vi "m100RecipeToExcelNew.vi"() -> ()   [LabVIEW 2012]
uses:
  <vilib>/addons/database/Auxilliary.llb/DB Tools Cursor Type.ctl
  <vilib>/Utility/NIReport.llb/NI_report.lvclass
  <vilib>/addons/database/Connection.llb/DB Tools Open Connec (Path).vi
  <vilib>/addons/database/Connection.llb/Conn Execute.vi
  <vilib>/addons/database/Recordset.llb/Rec Fetch Recordset Data (R).vi
  <vilib>/addons/database/Recordset.llb/Rec Destroy - Connection.vi
  <vilib>/Utility/NIReport.llb/Append Text Table to Report (wrap).vi
  <vilib>/addons/database/_DB Variant To Data/Database Variant To Data.xnode
  <vilib>/Utility/NIReport.llb/Excel/NI_Excel.lvclass
  <vilib>/addons/database/NI_Database_API.lvlib
panel:
  in  "template (empty)":path=path "O:/Monitor/Recipe/PTSE/Module_Recipe Mapping Table.xls"
  out "appended path":path
  out "error out 4":errorcluster
  out "recordset data":variant[][](array[variant])
  out "error out":errorcluster
  in  "Report Template":path=path "O:/Monitor/Report/Module_Recipe Mapping Table.xls"
  in  "Table Control":string[][](table)
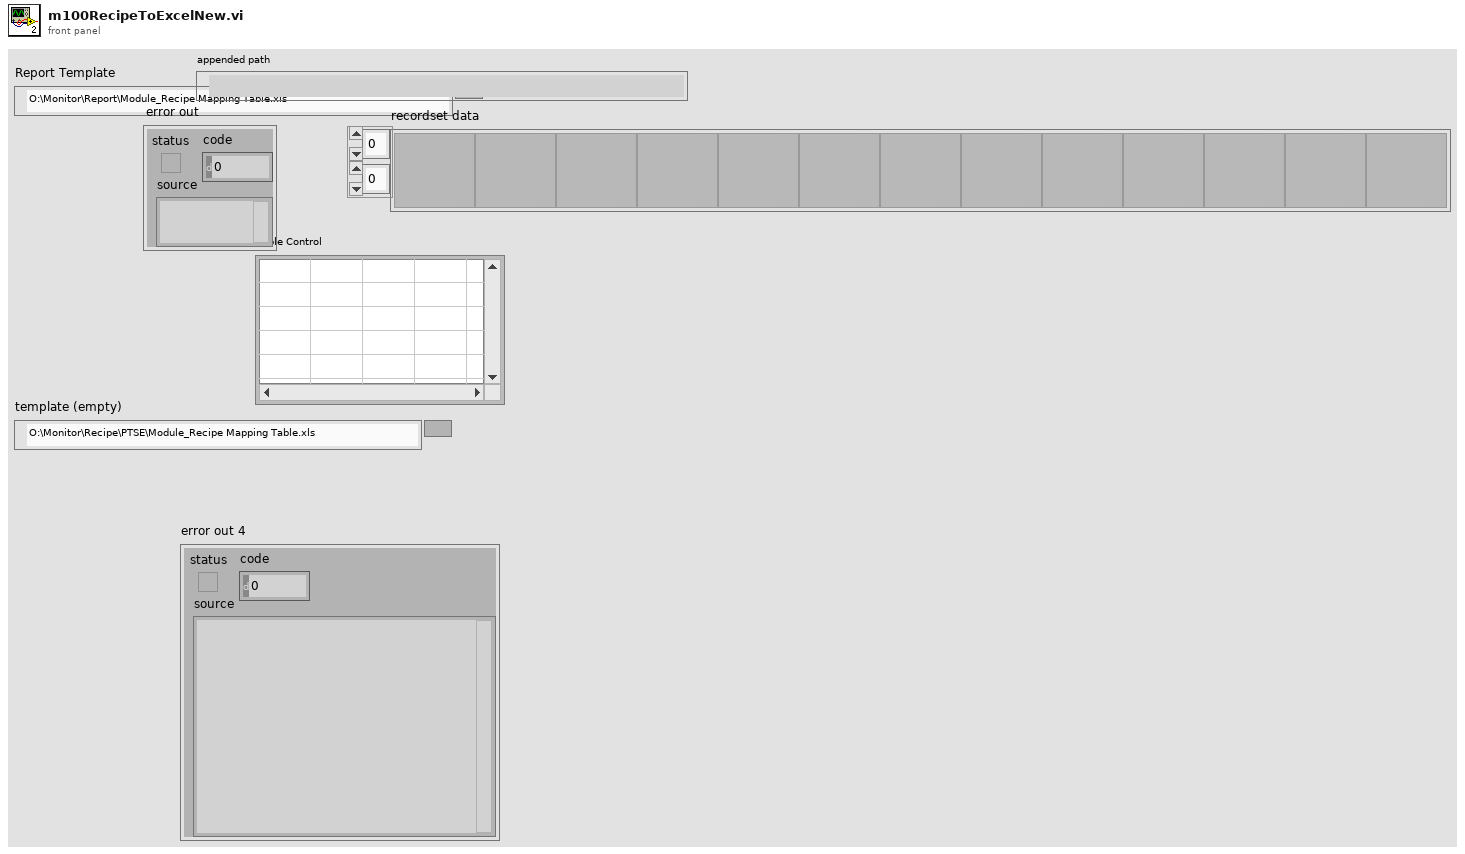
[diagram p1: front panel]
types:
  T1 = typedef "NI_Database_API.lvlib/DB Tools Cursor Type.ctl" = enum16{"forward-only", "keyset", "dynamic", "static"}
  T2 = typedef "NI_Database_API.lvlib/Conn ObjectReference.ctl" = refnum<k1>
  T3 = typedef "NI_Database_API.lvlib/Rec ObjectReference.ctl" = refnum<k1>
  T4 = enum16{"Standard Report", "HTML", "Word", "Excel"}
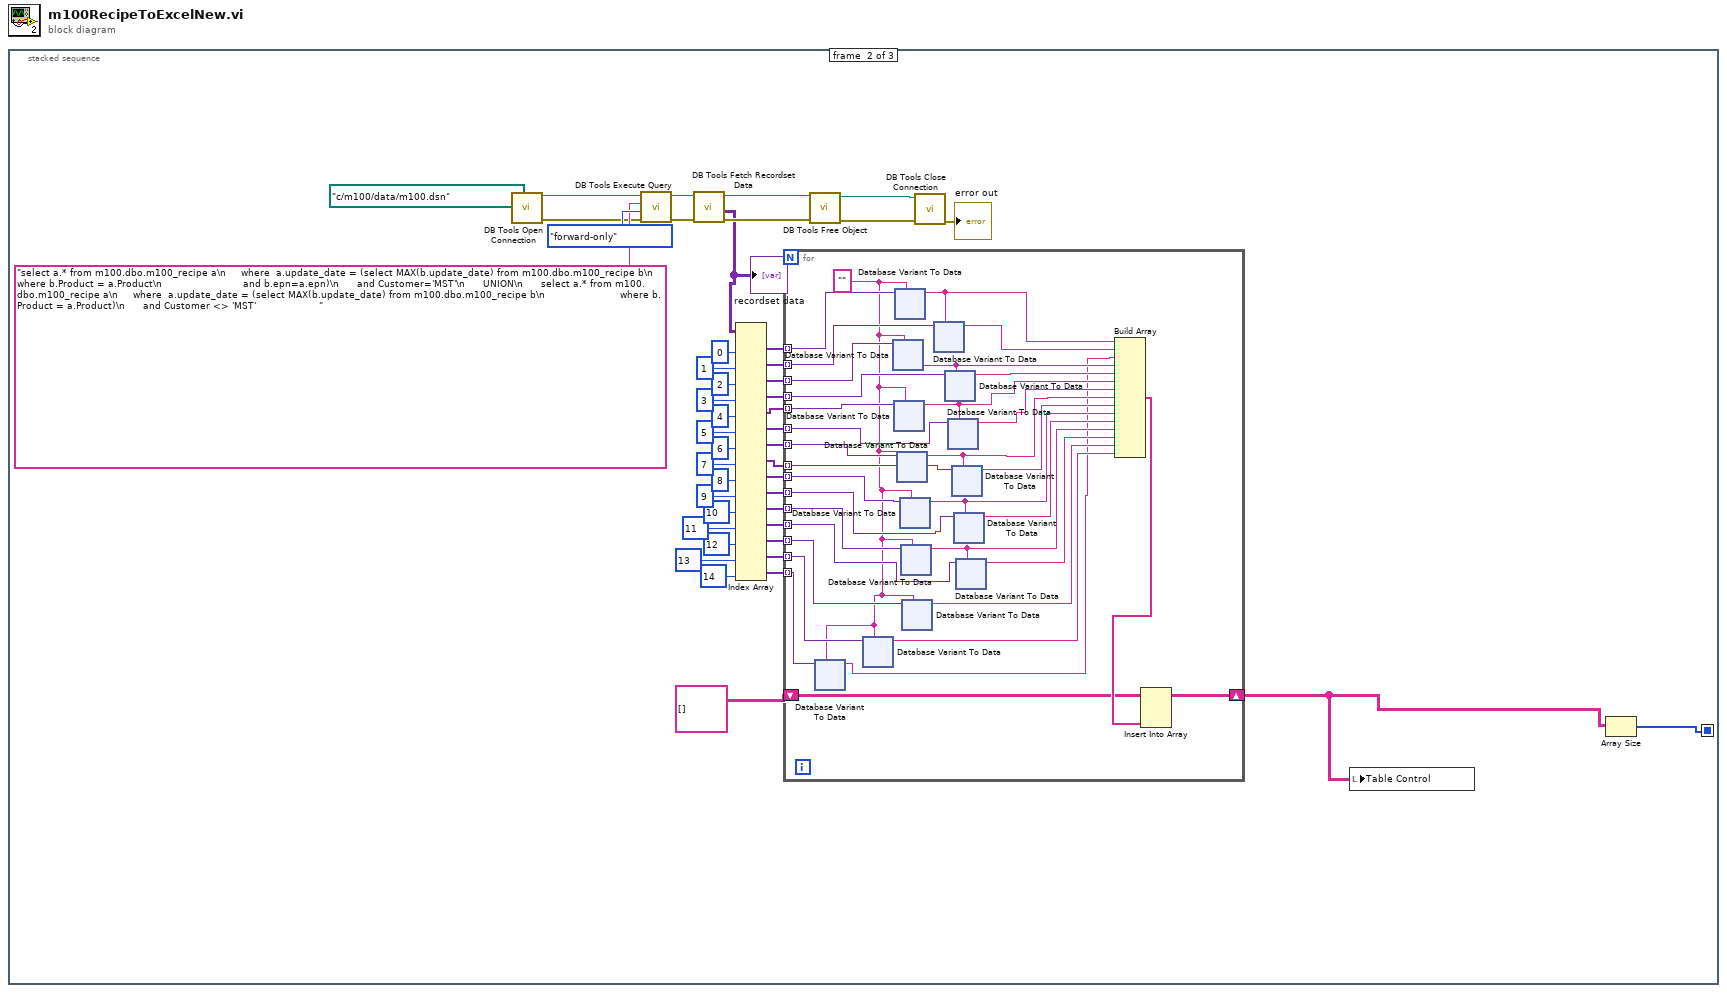
[diagram p0: block diagram]
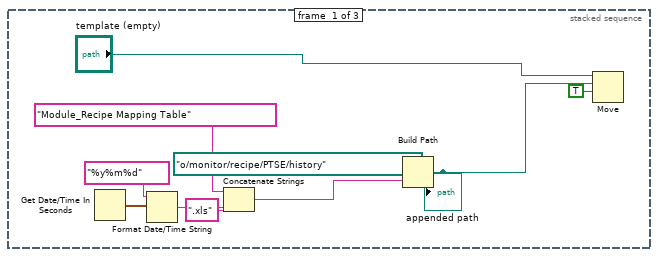
[diagram p2: hidden frame]
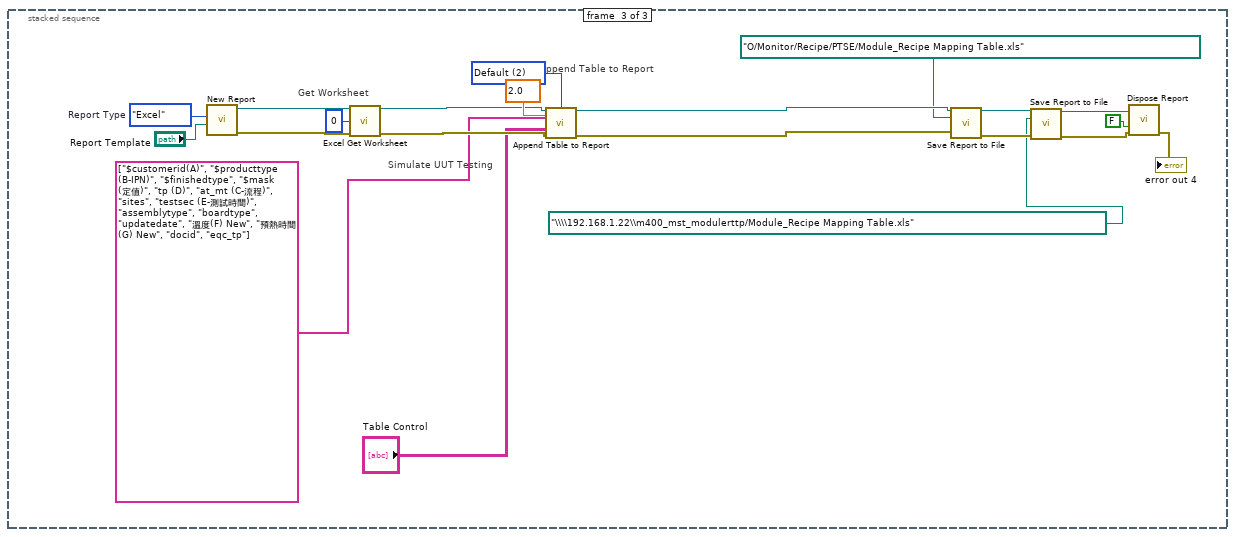
[diagram p3: hidden frame]
diagram:
  n1 = stacked-sequence {
    seq-local: [_ w56 _] -> [_ _ _]
    frame #0 {
      n2 = Get Date/Time In Seconds() -> (seconds since 1Jan1904=w8:timestamp)
      n3 = Format Date/Time String(time format string (%c)="%y%m%d", seconds (now)=w8) -> (date/time string=w6:string)  [unwired: 1 in]
      n4 = Concatenate Strings("Module_Recipe Mapping Table" ("string"), w6, ".xls" ("string")) -> (w9:string)
      n5 = Build Path(base path=path "o:/monitor/recipe/PTSE/history", name or relative path=w9) -> (appended path=w3:path)
      "appended path" <- w3
      n6 = Move(source path="template (empty)", 9:TRUE ("overwrite (F)"), 10:w3) -> ()  [unwired: 2 in, 3 out]
    }
    frame #1 {
      n7 = call-poly <vilib>:"DB Tools Open Connection.vi"("connection information"=path "c:/m100/data/m100.dsn") -> ("error out"=w23:errorcluster, "connection reference"=w24:T2)  [unwired: 7 in]
      n8 = call-poly <vilib>:"DB Tools Execute Query.vi"("error in (no error)"=w23, "cursor type"=DB_Tools_Cursor_Type."forward-only", "SQL query"="select a.* from m100.dbo.m100_recipe a\n     where  a.update_date = (select MAX(b.update_date) from m100.dbo.m100_recipe b\n                         where b.Product = a.Product\n                           and b.epn=a.epn)\n      and Customer='MST'\n      UNION\n      select a.* from m100.dbo.m100_recipe a\n     where  a.update_date = (select MAX(b.update_date) from m100.dbo.m100_recipe b\n                         where b.Product = a.Product)\n      and Customer <> 'MST'                     ", "connection reference"=w24) -> ("error out"=w55:errorcluster, "recordset reference"=w54:T3)  [unwired: 4 in]
      n9 = call-poly <vilib>:"DB Tools Fetch Recordset Data.vi"("error in (no error)"=w55, "recordset reference"=w54) -> ("error out"=w52:errorcluster, "recordset data"=w50:variant[][], "recordset reference out"=w53:T3)  [unwired: 3 in]
      "recordset data" <- w50
      n10 = Index Array(array=w50, index (col) #1=0 ("disabled index (col)"), index (col) #2=1 ("index (col)"), index (col) #3=2 ("index (col)"), index (col) #4=3 ("index (col)"), index (col) #5=4 ("index (col)"), index (col) #6=5 ("index (col)"), index (col) #7=6 ("index (col)"), index (col) #8=7 ("index (col)"), index (col) #9=8 ("index (col)"), index (col) #10=9 ("index (col)"), index (col) #11=10 ("index (col)"), index (col) #12=11 ("index (col)"), index (col) #13=12 ("index (col)"), index (col) #14=13 ("index (col)"), index (col) #15=14 ("index (col)")) -> (element #1=w47:variant[], element #2=w46:variant[], element #3=w45:variant[], element #4=w34:variant[], element #5=w33:variant[], element #6=w32:variant[], element #7=w31:variant[], element #8=w30:variant[], element #9=w29:variant[], element #10=w28:variant[], element #11=w27:variant[], element #12=w26:variant[], element #13=w17:variant[], element #14=w13:variant[], element #15=w11:variant[])  [unwired: 15 in]
      n11 = for {
        tunnel: w47 -> [w90] mode=indexing
        tunnel: w46 -> [w89] mode=indexing
        tunnel: w45 -> [w88] mode=indexing
        tunnel: w34 -> [w87] mode=indexing
        tunnel: w33 -> [w84] mode=indexing
        tunnel: w32 -> [w82] mode=indexing
        tunnel: w31 -> [w80] mode=indexing
        tunnel: w30 -> [w77] mode=indexing
        tunnel: w29 -> [w76] mode=indexing
        tunnel: w28 -> [w75] mode=indexing
        tunnel: w27 -> [w72] mode=indexing
        tunnel: w26 -> [w71] mode=indexing
        tunnel: w17 -> [w68] mode=indexing
        shift-right: [w65] -> w15
        shift-left: string[][] [] ("array") -> [w64]
        tunnel: w13 -> [w63] mode=indexing
        tunnel: w11 -> [w61] mode=indexing
        w60 = ""
        n12 = xnode "Database Variant To Data"("database variant"=w61, "type"=w60) -> ("data"=w57:string)  [unwired: 1 in, 1 out]
        n13 = xnode "Database Variant To Data"("database variant"=w63, "type"=w60) -> ("data"=w62:string)  [unwired: 1 in, 1 out]
        n14 = xnode "Database Variant To Data"("database variant"=w88, "type"=w60) -> ("data"=w86:string)  [unwired: 1 in, 1 out]
        n15 = xnode "Database Variant To Data"("database variant"=w84, "type"=w60) -> ("data"=w83:string)  [unwired: 1 in, 1 out]
        n16 = xnode "Database Variant To Data"("database variant"=w90, "type"=w60) -> ("data"=w59:string)  [unwired: 1 in, 1 out]
        n17 = xnode "Database Variant To Data"("database variant"=w80, "type"=w60) -> ("data"=w79:string)  [unwired: 1 in, 1 out]
        n18 = xnode "Database Variant To Data"("database variant"=w76, "type"=w60) -> ("data"=w74:string)  [unwired: 1 in, 1 out]
        n19 = xnode "Database Variant To Data"("database variant"=w72, "type"=w60) -> ("data"=w70:string)  [unwired: 1 in, 1 out]
        n20 = xnode "Database Variant To Data"("database variant"=w68, "type"=w60) -> ("data"=w67:string)  [unwired: 1 in, 1 out]
        n21 = xnode "Database Variant To Data"("database variant"=w89, "type"=w59) -> ("data"=w58:string)  [unwired: 1 in, 1 out]
        n22 = xnode "Database Variant To Data"("database variant"=w87, "type"=w86) -> ("data"=w85:string)  [unwired: 1 in, 1 out]
        n23 = xnode "Database Variant To Data"("database variant"=w82, "type"=w83) -> ("data"=w81:string)  [unwired: 1 in, 1 out]
        n24 = xnode "Database Variant To Data"("database variant"=w77, "type"=w79) -> ("data"=w78:string)  [unwired: 1 in, 1 out]
        n25 = xnode "Database Variant To Data"("database variant"=w75, "type"=w74) -> ("data"=w73:string)  [unwired: 1 in, 1 out]
        n26 = xnode "Database Variant To Data"("database variant"=w71, "type"=w70) -> ("data"=w69:string)  [unwired: 1 in, 1 out]
        n27 = Build Array(w59, w58, w57, w86, w85, w83, w81, w79, w78, w74, w73, w70, w69, w67, w62) -> (w66:string[])
        n28 = Insert Into Array(array=w64, new element=w66) -> (w65:string[][])  [unwired: 2 in]
      }
      n29 = call-poly <vilib>:"DB Tools Free Object.vi"("error in (no error)"=w52, "recordset reference"=w53) -> ("error out"=w20:errorcluster, "connection reference"=w21:T2)  [unwired: 8 in]
      n30 = call <vilib>:"DB Tools Close Connection.vi"("error in (no error)"=w20, "connection reference"=w21) -> ("error out"=→"error out":errorcluster)  [unwired: 5 in]
      n31 = local write "Table Control"(w15) -> ()
      n32 = Array Size(array=w15) -> (size(s)=w56:i32[])
    }
    frame #2 {
      w582 = u16 2 items=["US", "Metric", "Default"] ("measurement system")
      w591 = T4."Excel"  # Report Type
      # "Simulate UUT Testing"
      # "Append Table to Report"
      # "Get Worksheet"
      n33 = call <vilib>:"New Report.vi"("report type"=w591, "template (empty)"="Report Template") -> ("report out"=w588:refnum<class "NI_report.lvclass">, "error out"=w587:errorcluster)  [unwired: 12 in]
      n34 = call <vilib>:"Excel Get Worksheet.vi"("report in"=w588, "worksheet index (0)"=0, "error in (no error)"=w587) -> ("report out"=w586:refnum<class "NI_report.lvclass">, "error out"=w585:errorcluster)  [unwired: 11 in]
      n35 = call-poly <vilib>:"Append Table to Report.vi"("report in"=w586, "column width (1)"=2.0, "measurement system"=w582, "column headers"=string[] ["$customerid(A)", "$producttype (B-IPN)", "$finishedtype", "$mask (定值)", "tp (D)", "at_mt (C-流程)", "sites", "testsec (E-測試時間)", "assemblytype", "boardtype", "updatedate", "溫度(F) New", "預熱時間 (G) New", "docid", "eqc_tp"] ("row headers"), "text data"="Table Control", "error in (no error)"=w585) -> ("report out"=w574:refnum<class "NI_report.lvclass">, "error out"=w573:errorcluster)  [unwired: 6 in, 2 out]
      n36 = call-dynamic "Save Report to File.vi"("report in"=w574, "report file path"=path "O:/Monitor/Recipe/PTSE/Module_Recipe Mapping Table.xls", "error in (no error)"=w573) -> ("report out"=w578:refnum<class "NI_report.lvclass">, "error out"=w575:errorcluster)  [unwired: 11 in]
      n37 = call-dynamic "Save Report to File.vi"("report in"=w578, "report file path"=path "\\\\192.168.1.22\\m400_mst_modulerttp/Module_Recipe Mapping Table.xls", "error in (no error)"=w575) -> ("report out"=w577:refnum<class "NI_report.lvclass">, "error out"=w576:errorcluster)  [unwired: 11 in]
      n38 = call-dynamic "Dispose Report.vi"("report in"=w577, "save changes? (F)"=FALSE, "error in (no error)"=w576) -> ("error out"=→"error out 4":errorcluster)  [unwired: 12 in]
    }
  }
